vi "test.vi"() -> ()   [LabVIEW 2013]
panel:
  out "error out":errorcluster
  in  "错误输入（无错误）":errorcluster
  in  "VI名称或相对路径":string
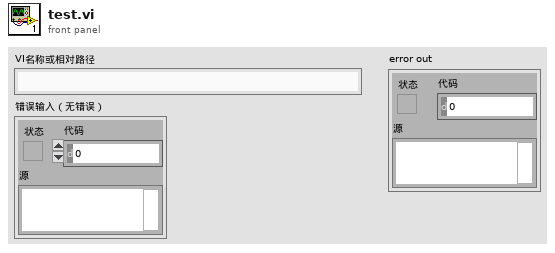
[diagram p1: front panel]
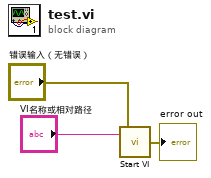
[diagram p0: block diagram]
diagram:
  n1 = call "Start VI.vi"("错误输入（无错误）"="错误输入（无错误）", "VI名称或相对路径"="VI名称或相对路径") -> ("error out"=→"error out":errorcluster)
